vi "Read Key DBL.vi"(7 "Section Name":string, 8 "error in":errorcluster, 9 "Default Value":dbl, 10 "Key Name":string, 11 "Config Cluster in":T1) -> (0 "error out":errorcluster, 1 "Value":dbl, 2 "Found?":bool, 3 "Config Cluster out":T1)   [LabVIEW 2017]
uses:
  Config Cluster.ctl
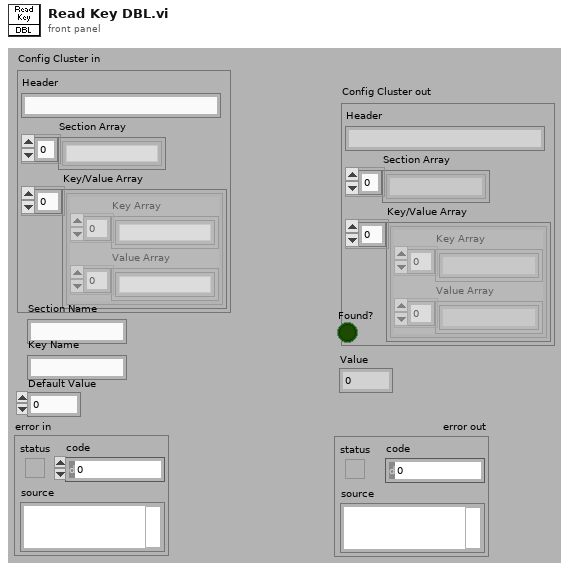
[diagram p1: front panel]
types:
  T1 = typedef "Config Cluster.ctl" = cluster{"Header":string, "Section Array":string[], "Key/Value Array":cluster{"Key Array":string[], "Value Array":string[]}[]}
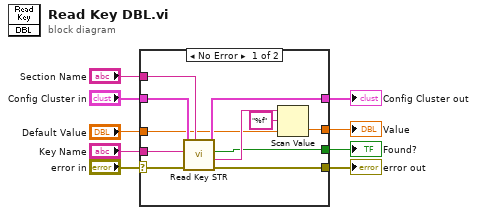
[diagram p0: block diagram]
diagram:
  n1 = case shown="No Error" "error in" {
    selector: "error in" -> [w20 w22]
    tunnel: [w19 w22] -> w8
    tunnel: "Config Cluster in" -> [w16 w23]
    tunnel: [w15 w23] -> w6
    tunnel: "Section Name" -> [w18 _]
    tunnel: "Key Name" -> [w17 _]
    tunnel: [w11 w21] -> w3
    tunnel: "Default Value" -> [w12 w21]
    tunnel: [w10 _] -> w1
    frame No Error {
      n2 = call "Read Key STR.vi"("Section Name"=w18, "error in"=w20, "Key Name"=w17, "Config Cluster in"=w16) -> ("error out"=w19:errorcluster, "Value"=w13:string, "Found?"=w10:bool, "Config Cluster out"=w15:T1)  [unwired: 4 in]
      n3 = Scan Value(string=w13, format string="%f", default (0 dbl)=w12) -> (value=w11:dbl)  [unwired: 1 out]
    }
    frame Error {
    }
  }
  "error out" <- w8
  "Config Cluster out" <- w6
  "Value" <- w3
  "Found?" <- w1
